vi "Temperature Warnings.vi"(8 "Error In":errorcluster, 11 "Weather Data In.":T1={"Current Temperature"=0.0, "Max Temperature"=0.0, "Min Temperature"=0.0, "Temperature Warning?"=FALSE, "Temperature Warning Text"="No Warning"}) -> (0 "Error Out":errorcluster, 3 "Weather Data Out.":T1={"Current Temperature"=0.0, "Max Temperature"=0.0, "Min Temperature"=0.0, "Temperature Warning?"=FALSE, "Temperature Warning Text"="No Warning"})   [LabVIEW 2017]
doc: "This VI is used to determine the string to output to the weather station based on the current temperature and limit settings.\n\nInputs: Current Temperature (DBL), Minimum Temperature (DBL), and Maximum Temperature (DBL).\nOutputs: Warning Text (string) and Warning? (Boolean)."
uses:
  Weather Station/Supporting Files/Weather Data.ctl
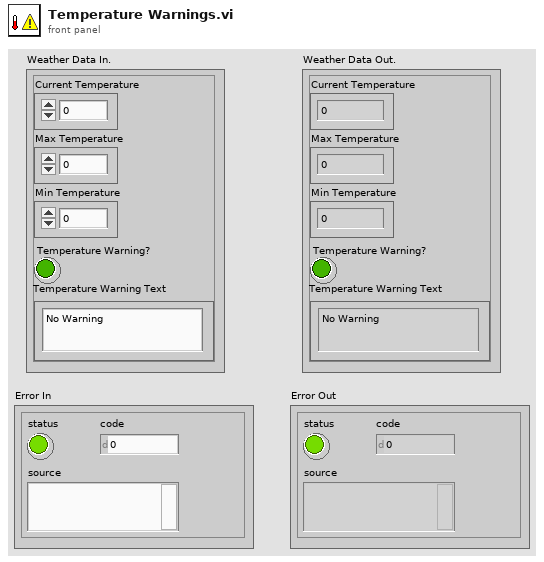
[diagram p1: front panel]
types:
  T1 = typedef "Weather Data.ctl" = cluster{"Current Temperature":dbl, "Max Temperature":dbl, "Min Temperature":dbl, "Temperature Warning?":bool, "Temperature Warning Text":string}
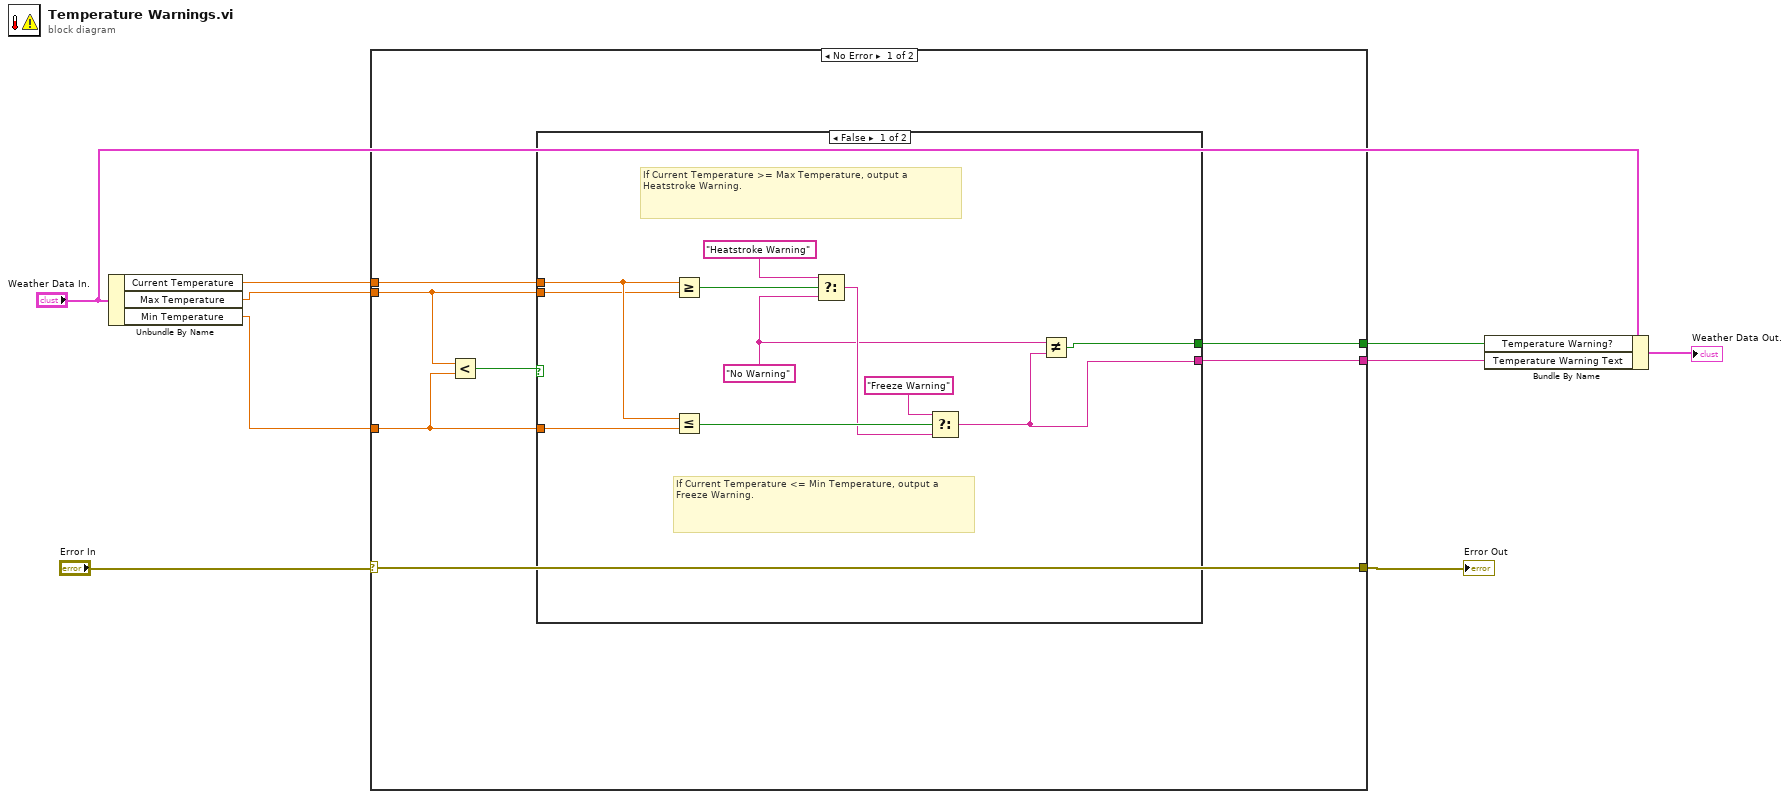
[diagram p0: block diagram]
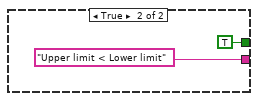
[diagram p2: hidden frame]
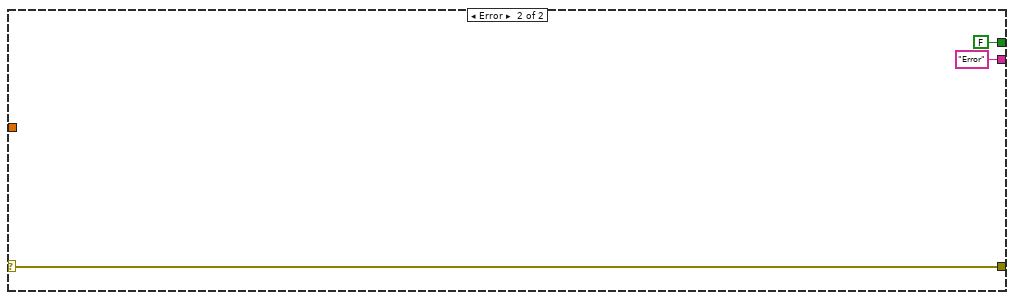
[diagram p3: hidden frame]
diagram:
  n1 = Unbundle By Name("Weather Data In.") -> ("Current Temperature"=w9:dbl, "Max Temperature"=w8:dbl, "Min Temperature"=w7:dbl)
  n2 = case shown="No Error" "Error In" {
    selector: "Error In" -> [w13 w32]
    tunnel: w9 -> [w16 _]
    tunnel: w8 -> [w12 _]
    tunnel: w7 -> [w11 _]
    tunnel: [w15 FALSE] -> w5
    tunnel: [w14 "Error" ("f")] -> w4
    tunnel: [w13 w32] -> w1
    frame No Error {
      n3 = Less?(x=w12, y=w11) -> (x < y?=w10:bool)
      n4 = case shown="False" w10 {
        tunnel: w16 -> [w21 _]
        tunnel: w12 -> [w20 _]
        tunnel: w11 -> [w19 _]
        tunnel: [w18 TRUE] -> w15
        tunnel: [w17 "Upper limit < Lower limit" ("f")] -> w14
        frame False {
          w22 = "No Warning" ("f")
          # "If Current Temperature >= Max Temperature, output a Heatstroke Warning."
          # "If Current Temperature <= Min Temperature, output a Freeze Warning."
          n5 = Greater Or Equal?(x=w21, y=w20) -> (x >= y?=w27:bool)
          n6 = Less Or Equal?(x=w21, y=w19) -> (x <= y?=w24:bool)
          n7 = Select(t="Heatstroke Warning", s=w27, f=w22) -> (s? t:f=w23:string)
          n8 = Select(t="Freeze Warning", s=w24, f=w23) -> (s? t:f=w17:string)
          n9 = Not Equal?(x=w22, y=w17) -> (x != y?=w18:bool)
        }
        frame True {
        }
      }
    }
    frame Error {
    }
  }
  "Error Out" <- w1
  n10 = Bundle By Name(cluster="Weather Data In.", "Temperature Warning?"=w5, "Temperature Warning Text"=w4) -> (→"Weather Data Out.":T1)
